vi "Fetch.vi"   [LabVIEW 2016, in "Keithley DMM6500 DAQ6500 Series.lvlib"]
doc: "Retrieve data from instrument."
uses:
  Keithley DMM6500 DAQ6500 Series.lvlib
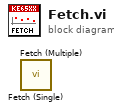
[diagram p0: block diagram]
diagram:
  n1 = call "Fetch (Single).vi"() -> ()  [unwired: 9 in, 3 out]
  n2 = call "Fetch (Multiple).vi"() -> ()  [unwired: 9 in, 3 out]
